vi "Post Submit.vi"(0 "Commit in":refnum<class "Commit.lvclass">) -> (4 "Commit out":refnum<class "Commit.lvclass">)   [LabVIEW 2017, in "CL_G3_VIComponentBuilder.lvlib" / "Commit.lvclass"]
doc: "All actions taken after comitting the export."
uses:
  Commit.lvclass
  Commit.lvclass/Commit.ctl
  Accessors/Read Commit Operation Errors.vi
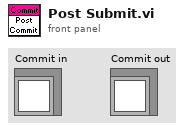
[diagram p1: front panel]
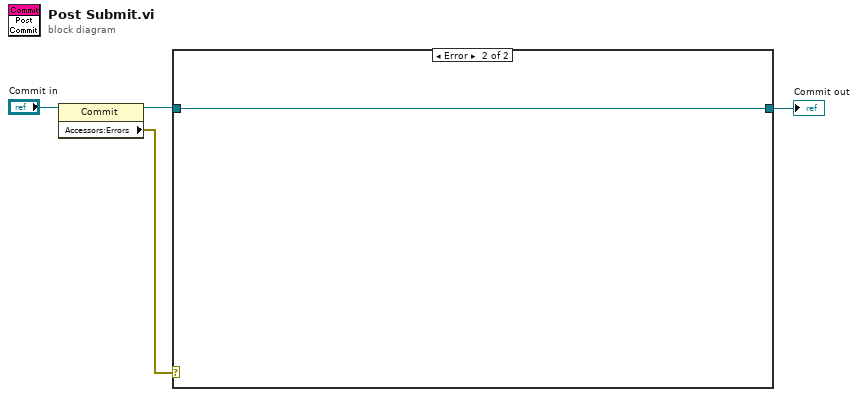
[diagram p0: block diagram]
diagram:
  n1 = property class="Commit"(reference="Commit in") -> (reference out=w2:refnum<class "Commit.lvclass">, "Accessors:Errors"=w1:errorcluster)  [unwired: 1 in, 1 out]
  n2 = case shown="Error" w1 {
    tunnel: [w5 w6] -> w4
    tunnel: w2 -> [w5 w6]
    frame No Error {
    }
    frame Error {
    }
  }
  "Commit out" <- w4
